vi "Format LV Error as JSON Data.vi"(10 "error in":errorcluster) -> (0 "error out":errorcluster, 2 "Error Object Out":refnum<class "JSON Object.lvclass">)   [LabVIEW 2015, in "JSONRPC Server.lvclass"]
doc: "This converts a LabVIEW Error to a JSON Tree for use with \"Add Response - Server Error\"."
uses:
  JSONRPC Server.lvclass
  <vilib>/NI/JSON Support for LabVIEW/JSON Data Classes/JSON Object/JSON Object.lvclass
  <vilib>/NI/JSON Support for LabVIEW/JSON Data Classes/JSON Object/New JSON Object (Empty).vi
  <vilib>/NI/JSON Support for LabVIEW/JSON Data Classes/JSON Object/Insert Key Value Pair (Single Numeric).vi
  <vilib>/NI/JSON Support for LabVIEW/JSON Data Classes/JSON Object/Insert Key Value Pair (Single String).vi
  <vilib>/NI/JSON Support for LabVIEW/JSON Data Classes/JSON Helper/JSON Helper.lvclass
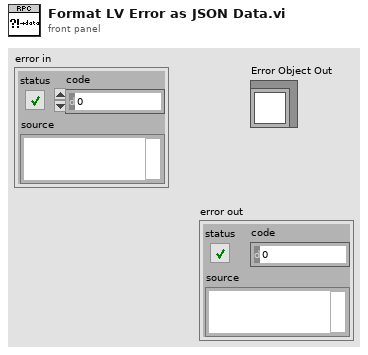
[diagram p1: front panel]
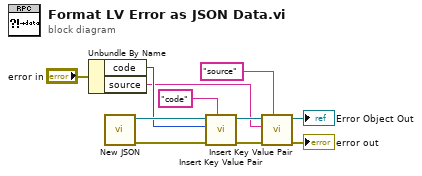
[diagram p0: block diagram]
diagram:
  n1 = Unbundle By Name("error in") -> ("code"=w4:i32, "source"=w2:string)
  n2 = call-poly <vilib>:"New JSON.vi"() -> ("error out"=w5:errorcluster, "JSON Object out"=w10:refnum<class "JSON Object.lvclass">)  [unwired: 10 in]
  n3 = call-poly <vilib>:"Insert Key Value Pair.vi"("key"="code" ("Name"), "error in (no error)"=w5, "value"=w4, "JSON Object in"=w10) -> ("error out"=w6:errorcluster, "JSON Object out"=w9:refnum<class "JSON Object.lvclass">)  [unwired: 5 in, 1 out]
  n4 = call-poly <vilib>:"Insert Key Value Pair.vi"("key"="source" ("Name"), "error in (no error)"=w6, "value"=w2, "JSON Object in"=w9) -> ("error out"=→"error out":errorcluster, "JSON Object out"=→"Error Object Out":refnum<class "JSON Object.lvclass">)  [unwired: 5 in, 1 out]
